vi "toOutput.vi"(6 "Chemin de sortie":path=path "C:/Users/manip/Documents/Thermo aquisition data/labview/output", 8 "Erreur en entrée":errorcluster caption="entrée d'erreur (pas d'erreur)", 9 "IP DAS240":string, 10 "Num de l'analyse":i32, 11 "Nom de l'analyse":string) -> (0 "Erreur en sortie":errorcluster caption="sortie d'erreur")   [LabVIEW 2019]
panel:
  out "chaîne concaténée":string
  out "standard error":string caption="erreur standard"
  out "standard output":string caption="sortie standard"
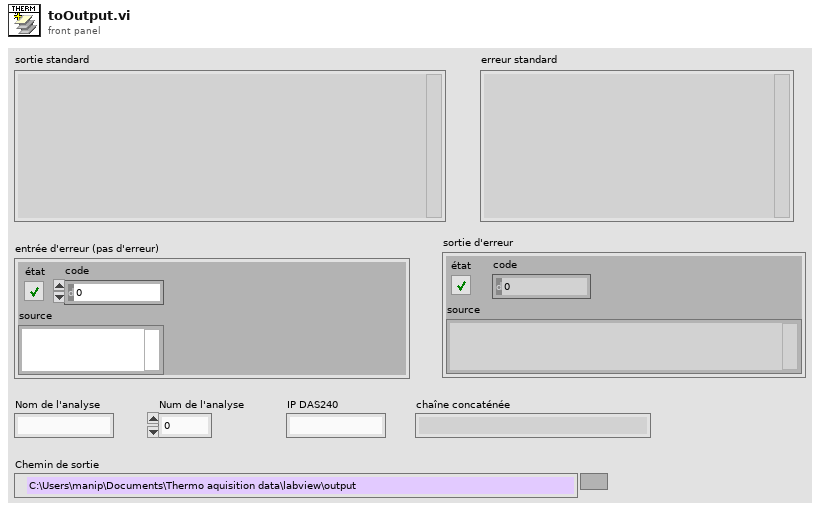
[diagram p1: front panel]
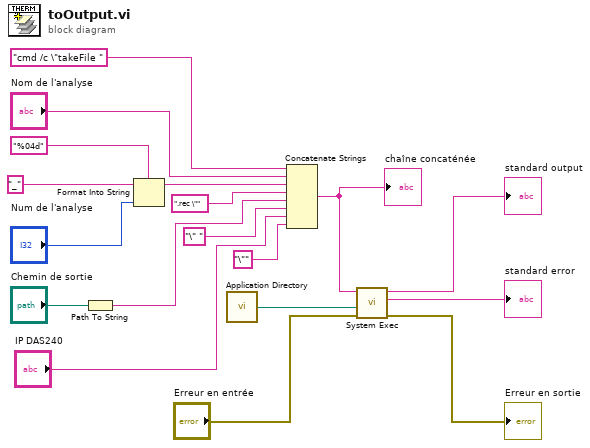
[diagram p0: block diagram]
diagram:
  n1 = Path To String(path="Chemin de sortie") -> (string=w4:string)
  n2 = Format Into String(format string="%04d" ("chaîne de format"), initial string="_" ("chaîne initiale"), "Num de l'analyse") -> (resulting string=w9:string)  [unwired: 1 in, 1 out]
  n3 = call <vilib>:"Application Directory.vi"() -> ("Application Directory"=w18:path)
  n4 = Concatenate Strings("cmd /c \"takeFile " ("chaîne"), "Nom de l'analyse", w9, ".rec \"" ("chaîne"), w4, "\" " ("chaîne"), "IP DAS240", "\"" ("chaîne")) -> (w6:string)
  "chaîne concaténée" <- w6
  n5 = call <vilib>:"System Exec.vi"("error in (no error)"="Erreur en entrée", "working directory"=w18, "command line"=w6) -> ("error out"=→"Erreur en sortie":errorcluster, "standard error"=→"standard error":string, "standard output"=→"standard output":string)  [unwired: 5 in, 1 out]
